vi "IHL_Wait for Motion Helper.vi"(5 "Status":u16 format="%x", 6 "EventLog ref":refnum<class "EventLog.lvclass">, 7 "Cancel":bool, 8 "error in (no error)":errorcluster, 9 "Loop Count in":i32, 10 "Next State":T1, 11 "Current State":T1) -> (0 "error out":errorcluster, 1 "Loop Count out":i32, 2 "Max Count Exceeded":bool, 3 "New State out":T1)   [LabVIEW 2015, in "Tool Module.lvlib"]
doc: "<b>Note:</b> This VI was modified by the <b>Validate DQMH Module</b> tool to turn off automatic error handling."
uses:
  Tool Module.lvlib
  _IHL SM Enum--typedef.ctl
  QC-X App/Libraries/Event Logger Library/Event Log/EventLog.lvclass
  ToolModGLOB.vi
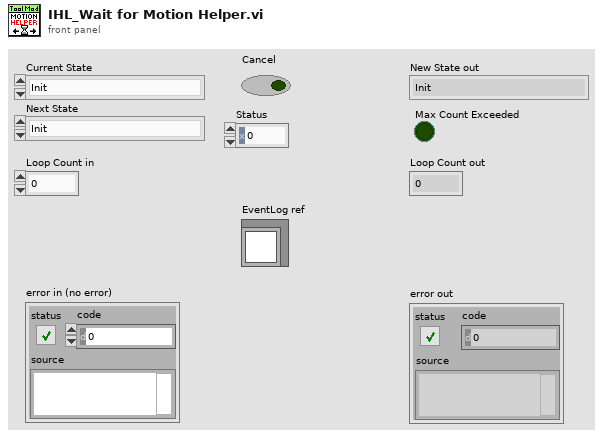
[diagram p1: front panel]
types:
  T1 = typedef "Tool Module.lvlib/_IHL SM Enum--typedef.ctl" = enum16{"Init", "Set Motion Speed", "Move To Scan Start", "Wait for Motion Out", "Wait for Start Pos", "Inspect: START", "Wait for Motion IN", "Wait for Inspect Range", "Inspecting", "Inspect: STOP"}
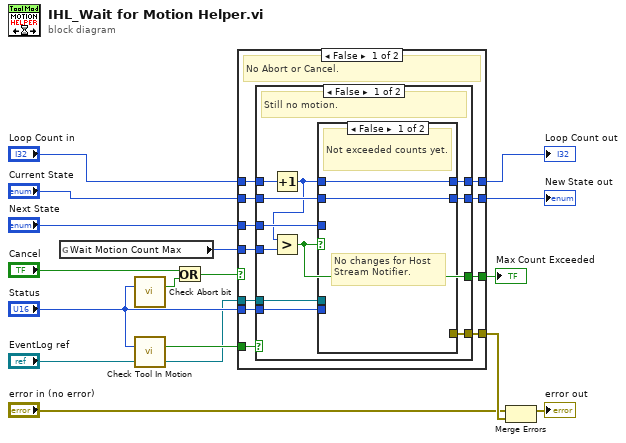
[diagram p0: block diagram]
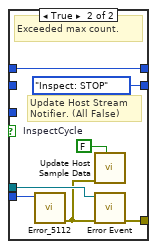
[diagram p2: hidden frame]
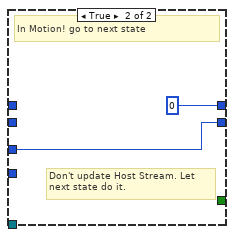
[diagram p3: hidden frame]
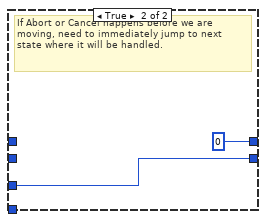
[diagram p4: hidden frame]
diagram:
  n1 = global read "ToolModGLOB.vi" "Wait Motion Count Max"() -> (w13:i32)
  n2 = call "Check Abort bit.vi"("Status Byte"="Status") -> ("Abort?"=w10:bool)  [unwired: 14 in]
  n3 = call "Check Tool In Motion.vi"("Status Byte"="Status") -> ("Tool In Motion?"=w16:bool)  [unwired: 14 in]
  n4 = Or(x="Cancel", y=w10) -> (x .or. y?=w8:bool)
  n5 = case shown="False" w8 {
    tunnel: w16 -> [w27 _]
    tunnel: [w26 w51] -> w15
    tunnel: "Next State" -> [w25 w51]
    tunnel: "Loop Count in" -> [w24 _]
    tunnel: w13 -> [w23 _]
    tunnel: "Status" -> [w22 _]
    tunnel: "Current State" -> [w21 _]
    tunnel: "EventLog ref" -> [w20 _]
    tunnel: [w19 0] -> w7
    tunnel: [w18 _] -> w6
    tunnel: [w17 _] -> w1
    frame False {
      # "No Abort or Cancel."
      n6 = case shown="False" w27 {
        tunnel: w24 -> [w38 _]
        tunnel: [w30 0] -> w19
        tunnel: w23 -> [w37 _]
        tunnel: w25 -> [w36 w48]
        tunnel: [w35 w48] -> w26
        tunnel: [w34 _] -> w18
        tunnel: w20 -> [w33 _]
        tunnel: w22 -> [w32 _]
        tunnel: w21 -> [w31 _]
        tunnel: [w29 _] -> w17
        frame False {
          # "Still no motion."
          n7 = Increment(x=w38) -> (x+1=w28:i32)
          n8 = Greater?(x=w28, y=w37) -> (0:w29:bool)
          n9 = case shown="False" w29 {
            tunnel: w36 -> [_ _]
            tunnel: [w40 _IHL_SM_Enum--typedef."Inspect: STOP" ("_Inspect SM Enum--typedef")] -> w35
            tunnel: [_ w46] -> w34
            tunnel: w33 -> [_ w45]
            tunnel: w32 -> [_ w44]
            tunnel: w31 -> [w40 _]
            tunnel: w28 -> [w39 w42]
            tunnel: [w39 w42] -> w30
            frame False {
              # "No changes for Host Stream Notifier."
              # "Not exceeded counts yet."
            }
            frame True {
              w41 = FALSE  # InspectCycle
              # "Update Host Stream Notifier. (All False)"
              # "Exceeded max count."
              n10 = call "Error_5112.vi"("Status Byte"=w44) -> ("error out"=w43:errorcluster)  [unwired: 10 in]
              n11 = call "Update Host Sample Data.vi"("InspectCycle"=w41, "error in (no error)"=w43) -> ()  [unwired: 9 in, 1 out]
              n12 = call "Error Event.vi"("error in (no error)"=w43, "EventLog ref"=w45) -> ("error out"=w46:errorcluster)  [unwired: 8 in, 1 out]
            }
          }
        }
        frame True {
          # "Don't update Host Stream. Let next state do it."
          # "In Motion! go to next state"
        }
      }
    }
    frame True {
      # "If Abort or Cancel happens before we are moving, need to immediately jump to next state where it will be handled."
    }
  }
  "New State out" <- w15
  "Loop Count out" <- w7
  "Max Count Exceeded" <- w1
  n13 = Merge Errors("error in (no error)", w6) -> (→"error out":errorcluster)
